vi "Cull and Group.vi"(8 "Min Compnt %":dbl=15.0, 9 "Score Cutoff %":dbl=70.0, 10 "Sorted Data":dbl[][](array[numeric]), 11 "Image Center":dbl) -> (2 "Best Targets above cutoff":T1(array[cluster]))   [LabVIEW 2018]
doc: "Examine the particle measurements to find the most likely pair that make up the target. This primarily compares the edges of the bounding boxes. It then returns information about the best two targets, notably the rectangle sourrounding the particles and the score."
panel:
  out "Grouping Scores":T2(array[cluster])
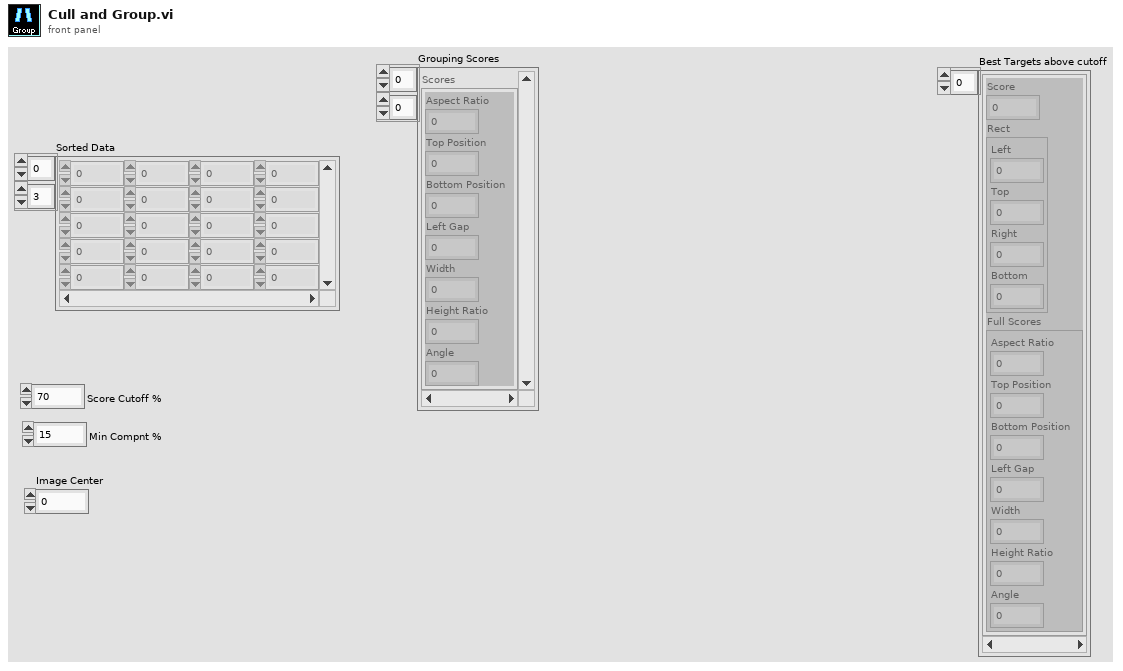
[diagram p1: front panel]
types:
  T1 = cluster{"Score":dbl, "Rect":cluster{"Left":dbl, "Top":dbl, "Right":dbl, "Bottom":dbl}, "Full Scores":cluster{"Aspect Ratio":dbl, "Top Position":dbl, "Bottom Position":dbl, "Left Gap":dbl, "Width":dbl, "Height Ratio":dbl, "Angle":dbl}}[]
  T2 = cluster{"Aspect Ratio":dbl, "Top Position":dbl, "Bottom Position":dbl, "Left Gap":dbl, "Width":dbl, "Height Ratio":dbl, "Angle":dbl}[][]
  T3 = cluster{"Left":dbl, "Top":dbl, "Right":dbl, "Bottom":dbl}
  T4 = cluster{"Aspect Ratio":dbl, "Strip Width":dbl, "Bottom Position":dbl, "Left Gap":dbl, "Width":dbl, "Height Ratio":dbl, "Angle":dbl}
  T5 = cluster{dbl, "Rect":cluster{"Left":dbl, "Top":dbl, "Right":dbl, "Bottom":dbl}, "Scores":cluster{"Aspect Ratio":dbl, "Strip Width":dbl, "Bottom Position":dbl, "Left Gap":dbl, "Width":dbl, "Height Ratio":dbl, "Angle":dbl}}
  T6 = cluster{dbl, "Rect":cluster{"Left":dbl, "Top":dbl, "Right":dbl, "Bottom":dbl}, "Scores":cluster{"Aspect Ratio":dbl, "Strip Width":dbl, "Bottom Position":dbl, "Left Gap":dbl, "Width":dbl, "Height Ratio":dbl, "Angle":dbl}}[]
  T7 = cluster{"Aspect Ratio":bool, "Strip Width":bool, "Bottom Position":bool, "Left Gap":bool, "Width":bool, "Height Ratio":bool, "Angle":bool}
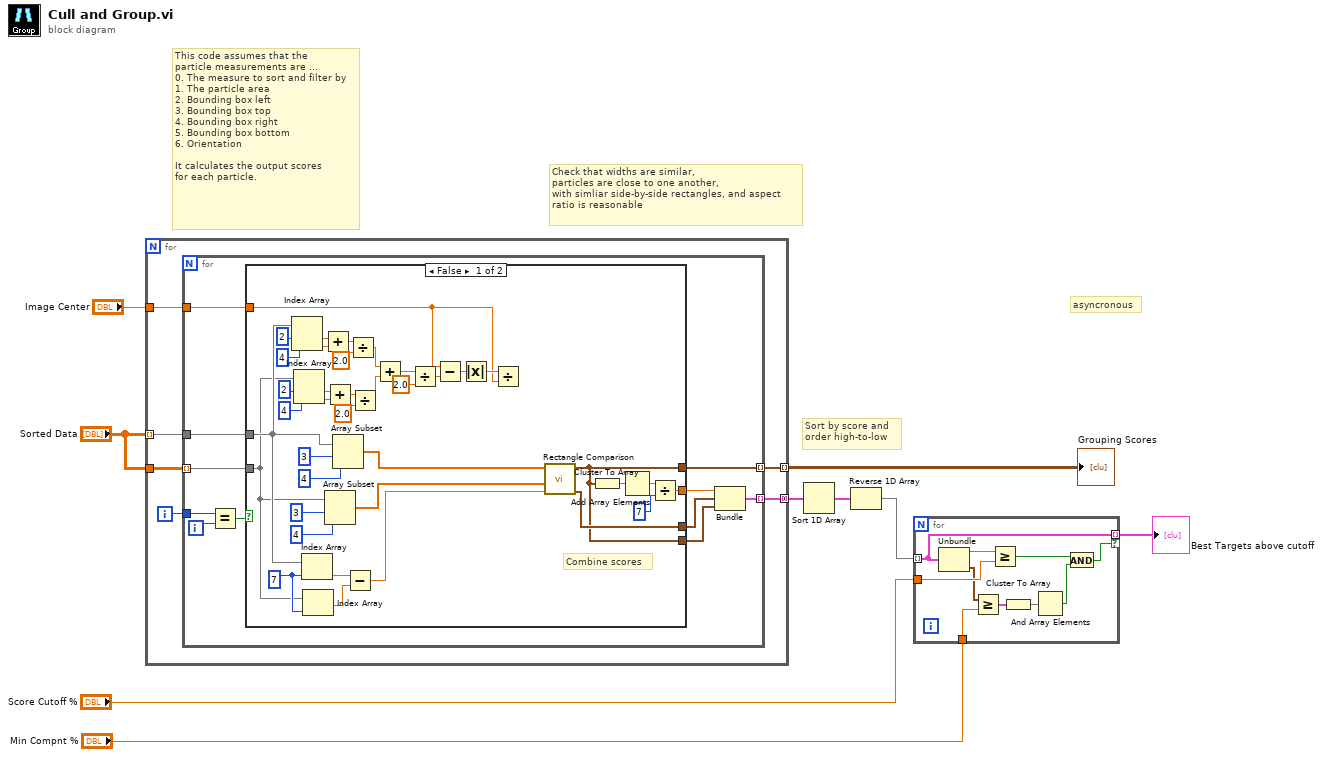
[diagram p0: block diagram]
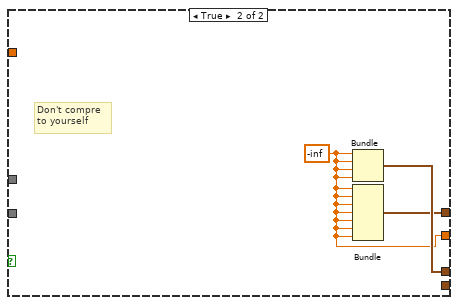
[diagram p2: hidden frame]
diagram:
  # "asyncronous"
  # "Sort by score and\norder high-to-low"
  # "Check that widths are similar,\nparticles are close to one another,\nwith simliar side-by-side rectangles, and aspect\nratio is reasonable"
  # "This code assumes that the\nparticle measurements are ...\n0. The measure to sort and filter by\n1. The particle area\n2. Bounding box left\n3. Bounding box top\n4. Bounding box right\n5. Bounding box bottom\n6. Orientation\n\nIt calculates the output scores\nfor each particle."
  n1 = for {
    tunnel: "Sorted Data" -> [w15] mode=indexing
    tunnel: "Sorted Data" -> [w14]
    tunnel: [w13] -> w9 mode=indexing
    tunnel: [w11] -> w7 mode=concatenating
    tunnel: "Image Center" -> [w10]
    i -> [w12]
    n2 = for {
      tunnel: w15 -> [w26]
      tunnel: w14 -> [w24] mode=indexing
      tunnel: [w16] -> w13 mode=indexing
      tunnel: w12 -> [w23]
      tunnel: [w19] -> w11 mode=indexing
      tunnel: w10 -> [w17]
      i -> [w22]
      n3 = Equal?(x=w23, y=w22) -> (x = y?=w25:bool)
      n4 = case shown="False" w25 {
        tunnel: w26 -> [w49 _]
        tunnel: w24 -> [w36 _]
        tunnel: [w54 w66] -> w21
        tunnel: [w57 w67] -> w20
        tunnel: [w27 _] -> w18
        tunnel: w17 -> [w28 _]
        tunnel: [w27 w65] -> w16
        frame False {
          w53 = 7 ("index")
          # "Combine scores"
          n5 = Index Array(array=w49, index #1=2 ("index"), index #2=4 ("index")) -> (element #1=w46:dbl, element #2=w45:dbl)
          n6 = Index Array(array=w36, index #1=2 ("index"), index #2=4 ("index")) -> (element #1=w39:dbl, element #2=w40:dbl)
          n7 = Index Array(array=w49, index=w53) -> (element=w52:dbl)
          n8 = Index Array(array=w36, index=w53) -> (element=w51:dbl)
          n9 = Add(x=w46, y=w45) -> (x+y=w44:dbl)
          n10 = Add(x=w39, y=w40) -> (x+y=w41:dbl)
          n11 = Array Subset(array=w36, index=3, length=4) -> (w58:dbl[])
          n12 = Array Subset(array=w49, index=3, length=4) -> (w59:dbl[])
          n13 = Subtract(x=w52, y=w51) -> (x-y=w50:dbl)
          n14 = Divide(x=w44, y=2.0) -> (x/y=w35:dbl)
          n15 = Divide(x=w41, y=2.0) -> (x/y=w34:dbl)
          n16 = Add(x=w35, y=w34) -> (x+y=w33:dbl)
          n17 = Divide(x=w33, y=2.0) -> (x/y=w31:dbl)
          n18 = Subtract(x=w28, y=w31) -> (x-y=w30:dbl)
          n19 = Absolute Value(x=w30) -> (abs(x)=w29:dbl)
          n20 = Divide(x=w29, y=w28) -> ()  [unwired: 1 out]
          n21 = call "Rectangle Comparison.vi"("Angle (deg)"=w50, "Second"=w58, "First"=w59) -> ("Rect"=w57:T3, "Scores"=w27:T4)  [unwired: 7 in]
          n22 = Cluster To Array(cluster=w27) -> (array=w60:dbl[])
          n23 = Add Array Elements(numeric array=w60) -> (sum=w55:dbl)
          n24 = Divide(x=w55, y=7 ("length")) -> (x/y=w54:dbl)
        }
        frame True {
          w66 = -inf
          # "Don't compre\nto yourself"
          n25 = Bundle(w66, w66, w66, w66) -> (w67:cluster{dbl, dbl, dbl, dbl})  [unwired: 1 in]
          n26 = Bundle(w66, w66, w66, w66, w66, w66, w66) -> (w65:cluster{dbl, dbl, dbl, dbl, dbl, dbl, dbl})  [unwired: 1 in]
        }
      }
      n27 = Bundle(w21, "Rect"=w20, "Scores"=w18) -> (w19:T5)  [unwired: 1 in]
    }
  }
  "Grouping Scores" <- w9
  n28 = Sort 1D Array(array=w7) -> (sorted array=w6:T6)
  n29 = Reverse 1D Array(array=w6) -> (reversed array=w5:T6)
  n30 = for {
    tunnel: w5 -> [w77] mode=indexing
    tunnel: [w77] -> w3 mode=indexing if=w68
    tunnel: "Score Cutoff %" -> [w75]
    tunnel: "Min Compnt %" -> [w73]
    n31 = Unbundle(w77) -> (w76:dbl, "Scores"=w74:T4)  [unwired: 1 out]
    n32 = Greater Or Equal?(x=w74, y=w73) -> (x >= y?=w72:T7)
    n33 = Greater Or Equal?(x=w76, y=w75) -> (x >= y?=w69:bool)
    n34 = Cluster To Array(cluster=w72) -> (array=w71:bool[])
    n35 = And Array Elements(Boolean array=w71) -> (logical AND=w70:bool)
    n36 = And(x=w69, y=w70) -> (x .and. y?=w68:bool)
  }
  "Best Targets above cutoff" <- w3
